vi "Setup APU.vi"   [LabVIEW 2013, in "APU.lvclass"]
uses:
  APU.lvclass
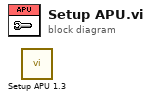
[diagram p0: block diagram]
diagram:
  n1 = call "Setup APU 1.3.vi"() -> ()  [unwired: 10 in, 2 out]
